vi "UMLEditor PostScriptTask.vi"(1 "ScriptFile":path, 2 "WaitForWiz":bool=TRUE, 5 "error in (no error)":errorcluster) -> (19 "error out":errorcluster)   [LabVIEW 2020]
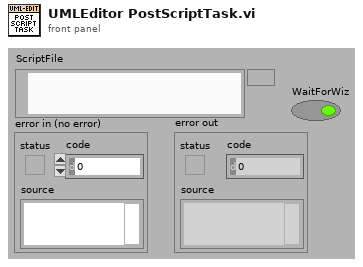
[diagram p1: front panel]
types:
  T1 = enum32{"Bad", "Idle", "Run top level", "Running"}
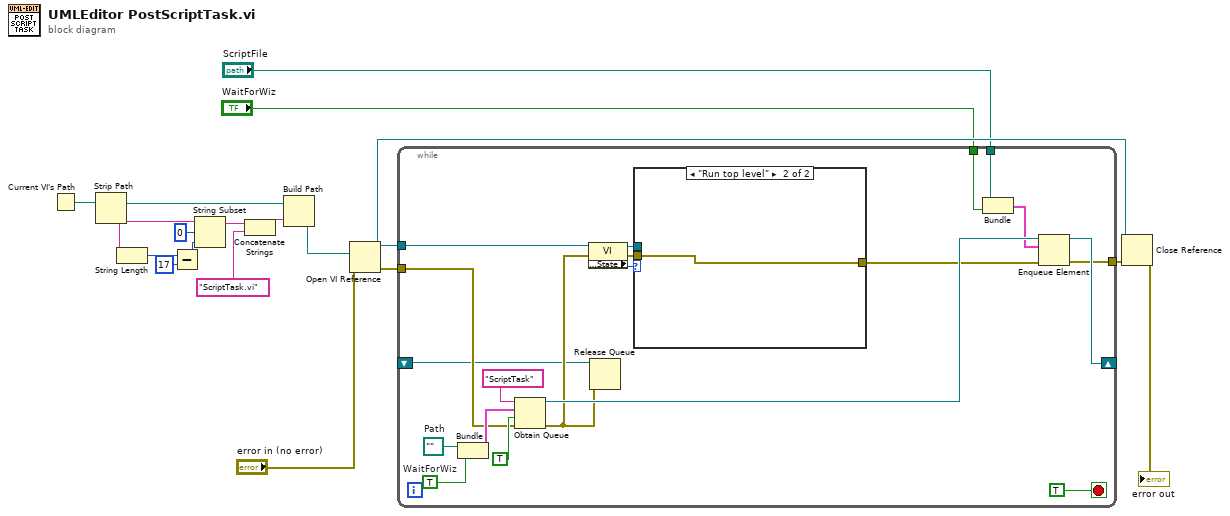
[diagram p0: block diagram]
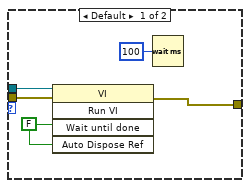
[diagram p2: hidden frame]
diagram:
  n1 = Current VI's Path() -> (path=w14:path)
  n2 = Strip Path(path=w14) -> (stripped path=w8:path, name=w13:string)
  n3 = String Length(string=w13) -> (length=w12:i32)
  n4 = Subtract(x=w12, y=17) -> (x-y=w10:i32)
  n5 = String Subset(string=w13, offset (0)=0, length (rest)=w10) -> (substring=w9:string)
  n6 = Concatenate Strings(w9, "ScriptTask.vi" ("string")) -> (w7:string)
  n7 = Build Path(base path=w8, name or relative path=w7) -> (appended path=w4:path)
  n8 = Open VI Reference(vi path=w4, error in (no error)="error in (no error)") -> (vi reference=w16:refnum<vi>, error out=w1:errorcluster)  [unwired: 4 out]
  n9 = while {
    tunnel: [w19] -> w17
    tunnel: w16 -> [w32]
    tunnel: "ScriptFile" -> [w28]
    tunnel: "WaitForWiz" -> [w27]
    tunnel: w1 -> [w25]
    shift-right: [w22] -> _
    shift-left: _ -> [w20]
    stop <- TRUE stop-if-true
    w30 = TRUE  # WaitForWiz
    w31 = path ""  # Path
    n10 = Bundle("Path"=w31, "WaitForWiz"=w30) -> (w29:cluster{"Path":path, "WaitForWiz":bool})  [unwired: 1 out]
    n11 = Obtain Queue(name (unnamed)="ScriptTask", element data type=w29, create if not found? (T)=TRUE, error in (no error)=w25) -> (queue out=w34:refnum<queue>, error out=w21:errorcluster)  [unwired: 1 in, 1 out]
    n12 = property class="VI"(reference=w32, error in=w21) -> (reference out=w33:refnum<vi>, error out=w36:errorcluster, "Execution:State"=w37:T1)
    n13 = Release Queue(queue=w20, error in (no error)=w21) -> ()  [unwired: 4 out]
    n14 = case shown="\"Run top level\"" w37 {
      tunnel: [w39 w44] -> w24
      tunnel: w36 -> [w42 w44]
      tunnel: w33 -> [w43 _]
      frame Default {
        w41 = FALSE ("Wait until done")
        n15 = invoke class="VI" method="Run VI"(reference=w43, error in=w42, "Wait until done"=w41, "Auto Dispose Ref"=w41) -> (error out=w39:errorcluster)  [unwired: 1 in, 4 out]
        n16 = Wait (ms)(milliseconds to wait=u32 100) -> ()  [unwired: 1 out]
      }
      frame "Run top level" {
      }
    }
    n17 = Bundle("ScriptFile"=w28, "WaitForWiz"=w27) -> (w26:cluster{"ScriptFile":path, "WaitForWiz":bool})  [unwired: 1 out]
    n18 = Enqueue Element(queue=w34, element=w26, error in (no error)=w24) -> (queue out=w22:refnum<queue>, error out=w19:errorcluster)  [unwired: 2 out]
  }
  n19 = Close Reference(reference=w16, error in (no error)=w17) -> (error out=→"error out":errorcluster)
